vi "Update-main-display.vi"(8 "error in":errorcluster, 10 "Data ref. in":refnum<data-value>, 11 "UI ref. in":refnum<data-value>) -> (0 "error IO":errorcluster, 2 "Data ref.":refnum<data-value>, 3 "UI ref.":refnum<data-value>)   [LabVIEW 2013, in "CameraVision.lvlib" / "CV-UI.lvclass"]
doc: "This function refreshes the main GUI display elements. These include currently the single camera view, the dual camera view, the analysis view (image, histogram and data tables), the temperature graph and the characteristic map graph.\nDuring an acquisition the active display is continuously updated (at 5 updates per second max.), unless the 'Image refresh' button is off. Outside of an acquisition the active display is only refreshed (once) when a display related parameter is changed (active display, display camera, display image, batch selector) or if the 'Image refresh' button is pressed. The function determines whether it is outside or inside an acquisition based on the 'Stop' notifier state (true = outside acquisition)."
uses:
  CV-UI.lvclass
  Main/CV-Main.lvclass
  CV-UI.lvclass/CV-UI.ctl
  Read Image refresh.vi
  Read Display-tab.vi
  Main/Errors/CV-Errors.lvclass
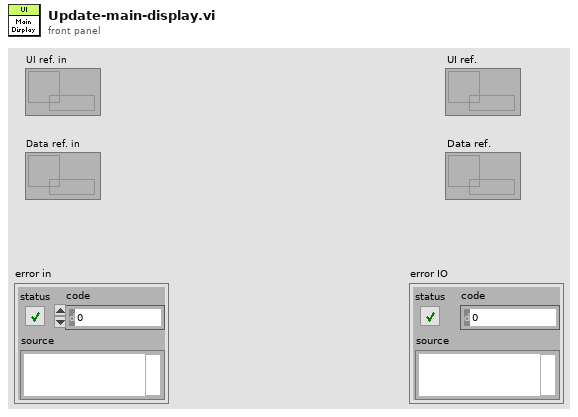
[diagram p1: front panel]
types:
  T1 = typedef "CameraVision.lvlib/CV-UI.lvclass/Display-selector.ctl" = enum32{"Single view", "Dual view", "Analysis", "History", "Temperature field", "Mapping", "Debug"}
  T2 = typedef "IMAQ Image.ctl" = refnum<image>
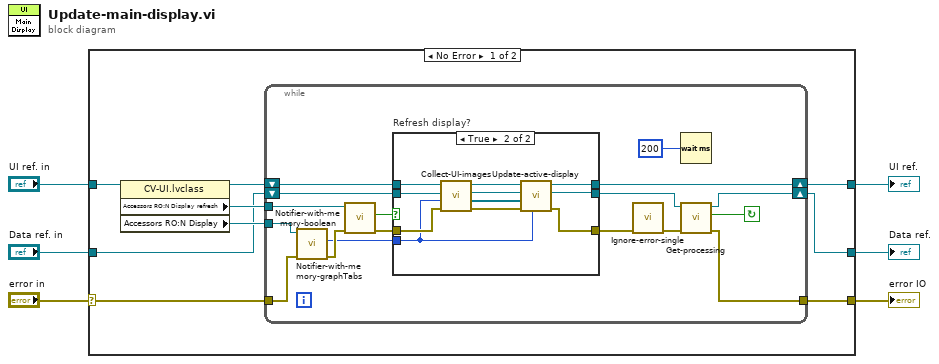
[diagram p0: block diagram]
diagram:
  n1 = case shown="No Error" "error in" {
    selector: "error in" -> [w14 w49]
    tunnel: "Data ref. in" -> [w8 w47]
    tunnel: "UI ref. in" -> [w15 w48]
    tunnel: [w13 w49] -> w3
    tunnel: [w10 w48] -> w1
    tunnel: [w7 w47] -> w2
    frame No Error {
      n2 = property class="CV-UI.lvclass"(reference=w15) -> (reference out=w11:refnum<data-value>, "Accessors RO:N Display refresh"=w12:refnum<notifier>, "Accessors RO:N Display"=w9:refnum<notifier>)  [unwired: 1 in, 1 out]
      n3 = while {
        tunnel: w12 -> [w25]
        shift-right: [w22] -> w10
        shift-left: w11 -> [w24]
        shift-right: [w21] -> w7
        shift-left: w8 -> [w23]
        tunnel: w9 -> [w16]
        tunnel: w14 -> [w19]
        tunnel: [w27] -> w13
        stop <- w26 continue-if-true
        n4 = call "Notifier-with-memory-graphTabs.vi"("error in"=w19, "Display-tab"=w16) -> ("error IO"=w18:errorcluster, "Notification"=w17:T1)  [unwired: 8 in]
        n5 = call "Notifier-with-memory-boolean.vi"("error in"=w18, "Notifier in"=w25) -> ("error IO"=w31:errorcluster, "Notification"=w32:bool)  [unwired: 8 in]
        n6 = case "Refresh display?" shown="True" w32 {
          tunnel: w31 -> [w35 w45]
          tunnel: [w35 w46] -> w29
          tunnel: w24 -> [w34 w44]
          tunnel: w23 -> [w33 w43]
          tunnel: [w34 w39] -> w22
          tunnel: [w33 w37] -> w20
          tunnel: w17 -> [_ w36]
          frame False {
          }
          frame True {
            n7 = call "Collect-UI-images.vi"("error in (no error)"=w45, "Active display"=w36, "Data ref. in"=w43, "UI ref. in in"=w44) -> ("error out"=w42:errorcluster, "Image refs"=w40:T2[], "Data ref."=w38:refnum<data-value>, "UI ref. out"=w41:refnum<data-value>)  [unwired: 4 in]
            n8 = call "Update-active-display.vi"("Active display"=w36, "error in (no error)"=w42, "Image refs"=w40, "Data ref. in"=w38, "UI ref. in"=w41) -> ("error out"=w46:errorcluster, "Data ref."=w37:refnum<data-value>, "UI ref."=w39:refnum<data-value>)  [unwired: 4 in]
          }
        }
        n9 = call "Ignore-error-single.vi"("error in (no error)"=w29) -> ("error out"=w28:errorcluster)  [unwired: 10 in]
        n10 = Wait (ms)(milliseconds to wait=u32 200 ("UI update interval")) -> ()  [unwired: 1 out]
        n11 = call "Get-processing.vi"("error in (no error)"=w28, "Data ref. in"=w20) -> ("error out"=w27:errorcluster, "Processing?"=w26:bool, "Data ref."=w21:refnum<data-value>)  [unwired: 7 in]
      }
    }
    frame Error {
    }
  }
  "error IO" <- w3
  "Data ref." <- w2
  "UI ref." <- w1
